vi "BuildHWI.vi"(8 "error in (no error)":errorcluster, 10 "Master Device in":refnum<class "Master Device.lvclass">, 11 "Arduino in":refnum<class "Arduino.lvclass">) -> (0 "error out":errorcluster, 2 "Master Device out":refnum<class "Master Device.lvclass">, 3 "Arduino out":refnum<class "Arduino.lvclass">)   [LabVIEW 2013, in "Arduino.lvclass"]
doc: "The previous subVI Prune.vi took the \"prepared\" private data and removed unnecessary points. Here in BuildHWI, one should turn the \"prepared\" data into a HWI that can be programmed to the physical device.\n (1) Flatten the data structure and put in normal time order"
uses:
  Arduino.lvclass
  Master Device/Master Device.lvclass
  Arduino.lvclass/Arduino.ctl
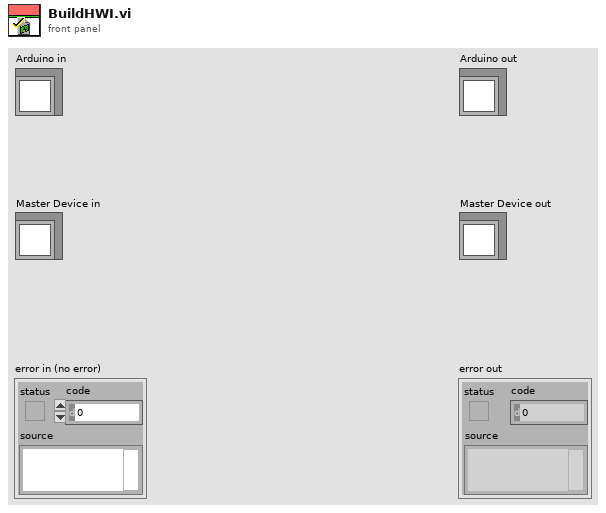
[diagram p1: front panel]
types:
  T1 = cluster{"Short Command":string, "ParamTotal":dbl, "Params":dbl[]}[][]
  T2 = cluster{"Short Command":string, "ParamTotal":dbl, "Params":dbl[]}[]
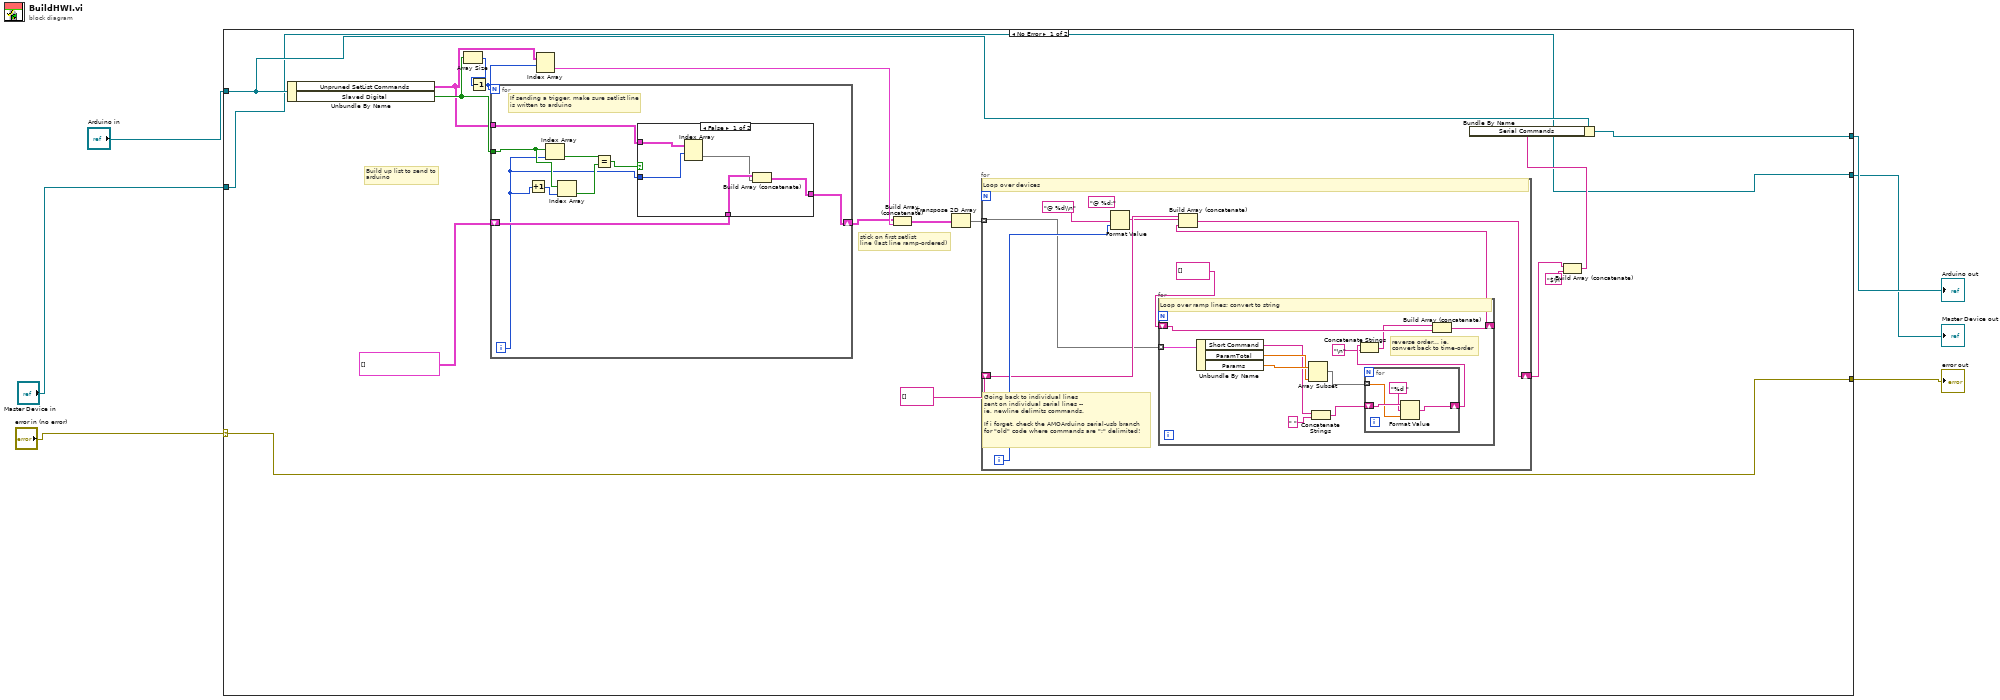
[diagram p0: block diagram]
diagram:
  n1 = case shown="No Error" "error in (no error)" {
    selector: "error in (no error)" -> [w9 w65]
    tunnel: [w9 w65] -> w1
    tunnel: [w7 w64] -> w2
    tunnel: "Master Device in" -> [w7 w64]
    tunnel: [w19 w63] -> w3
    tunnel: "Arduino in" -> [w8 w63]
    frame No Error {
      # "stick on first setlist\nline (last line ramp-ordered)"
      # "Build up list to send to\narduino"
      n2 = Unbundle By Name(w8) -> ("Unpruned SetList Commands"=w17:T1, "Slaved Digital"=w22:bool[])
      n3 = Array Size(array=w22) -> (size(s)=w18:i32)
      n4 = Decrement(x=w18) -> (x-1=w16:i32)
      n5 = for {
        N: w16 -> [_]
        tunnel: w17 -> [w49]
        tunnel: w22 -> [w55]
        shift-right: [w51] -> w14
        shift-left: T1 [] ("Unpruned SetList Commands") -> [w50]
        i -> [w48]
        # "If sending a trigger, make sure setlist line\nis written to arduino"
        n6 = Increment(x=w48) -> (x+1=w56:i32)
        n7 = Index Array(array=w55, index=w48) -> (element=w54:bool)
        n8 = Index Array(array=w55, index=w56) -> (element=w53:bool)
        n9 = Equal?(x=w54, y=w53) -> (x = y?=w52:bool)
        n10 = case shown="False" w52 {
          tunnel: [w60 w62] -> w51
          tunnel: w50 -> [w61 w62]
          tunnel: w49 -> [w59 _]
          tunnel: w48 -> [w58 _]
          frame False {
            n11 = Index Array(array=w59, index (row)=w58) -> (element=w57:T2)  [unwired: 1 in]
            n12 = Build Array (concatenate)(w61, w57) -> (w60:T1)
          }
          frame True {
          }
        }
      }
      n13 = Index Array(array=w17, index (row)=w16) -> (element=w15:T2)  [unwired: 1 in]
      n14 = Build Array (concatenate)(w14, w15) -> (w13:T1)
      n15 = Transpose 2D Array(2D array=w13) -> (transposed array=w21:T1)
      n16 = for {
        tunnel: w21 -> [w28] mode=indexing
        shift-right: [w25] -> w12
        shift-left: string[] [] -> [w30]
        i -> [w31]
        (unwired) "@ %d;"
        # "Going back to individual lines\nsent on individual serial lines -- \nie, newline delimits commands.\n\nIf i forget, check the AMOArduino serial-usb branch\nfor \"old\" code where commands are \";\" delimited!"
        # "Loop over devices"
        n17 = Format Value(format string="@ %d\\n", value (0)=w31) -> (output string=w29:string)  [unwired: 1 in]
        n18 = for {
          tunnel: w28 -> [w43] mode=indexing
          shift-right: [w38] -> w26
          shift-left: string[] [] ("appended array") -> [w35]
          # "reverse order... ie, \nconvert back to time-order"
          # "Loop over ramp lines; convert to string"
          n19 = Unbundle By Name(w43) -> ("Short Command"=w40:string, "ParamTotal"=w41:dbl, "Params"=w42:dbl[])
          n20 = Array Subset(array=w42, length=w41) -> (w37:dbl[])  [unwired: 1 in]
          n21 = Concatenate Strings(w40, " ") -> (w36:string)
          n22 = for {
            tunnel: w37 -> [w45] mode=indexing
            shift-right: [w44] -> w34
            shift-left: w36 -> [w47]
            n23 = Format Value(string ("")=w47, format string="%d ", value (0)=w45) -> (output string=w44:string)
          }
          n24 = Concatenate Strings(w34, "\n") -> (w33:string)
          n25 = Build Array (concatenate)(w33, w35) -> (w38:string[])
        }
        n26 = Build Array (concatenate)(w30, w29, w26) -> (w25:string[])
      }
      n27 = Build Array (concatenate)(w12, "$\n") -> (w10:string[])
      n28 = Bundle By Name(cluster=w8, "Serial Commands"=w10) -> (w19:refnum<class "Arduino.lvclass">)
    }
    frame Error {
    }
  }
  "error out" <- w1
  "Arduino out" <- w3
  "Master Device out" <- w2
